vi "Add Task.vi"(8 "error in (no error)":errorcluster, 10 "Task":refnum<class>, 11 "Work Dispatcher In":refnum<class "Work Dispatcher.lvclass">) -> (0 "error out":errorcluster, 3 "Work Dispatcher Out":refnum<class "Work Dispatcher.lvclass">)   [LabVIEW 2020, in "Work Dispatcher.lvclass"]
uses:
  Work Dispatcher.lvclass
  C:/Program Files (x86)/National Instruments/LabVIEW 2020/vi.lib/Asteme/Triarc Framework/Process/Process.lvclass
  <vilib>/Asteme/Triarc Framework/Process/Process.lvclass/Process.ctl
  <vilib>/Asteme/Triarc Framework/Process/Public/Lifecycle/Get Lifecycle State.vi
  <vilib>/Utility/error.llb/Clear Errors.vi
  <vilib>/Utility/error.llb/Error Cluster From Error Code.vi
  <vilib>/Asteme/Triarc Framework/Process/Process.lvclass
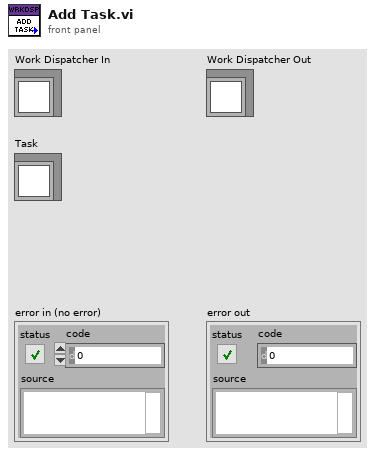
[diagram p1: front panel]
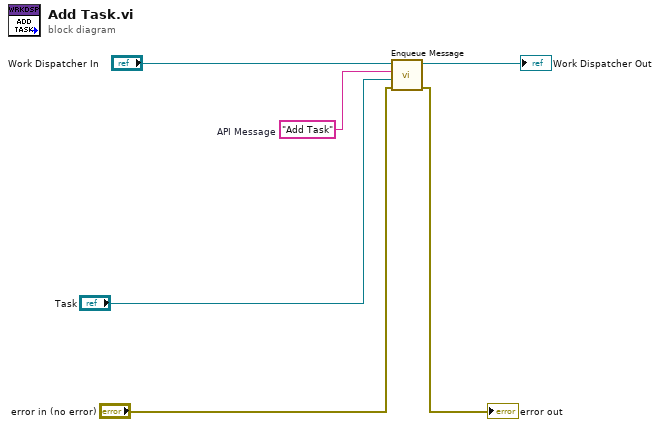
[diagram p0: block diagram]
diagram:
  w3 = "Add Task"  # API Message
  n1 = call <vilib>:"Enqueue Message.vi"("error in (no error)"="error in (no error)", "Message Data"="Task", "Message"=w3, "Process In"="Work Dispatcher In") -> ("error out"=→"error out":errorcluster, "Process Out"=→"Work Dispatcher Out":refnum<class "Work Dispatcher.lvclass">)  [unwired: 6 in]
